vi "Init.vi"(8 "error in (no error)":errorcluster, 10 "Message":T1, 11 "Queue in":refnum<queue>) -> (0 "error out":errorcluster, 3 "Queue out":refnum<queue>)   [LabVIEW 2016]
uses:
  Controls/Message Structure.ctl
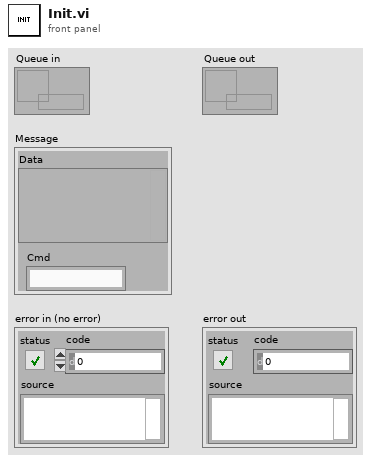
[diagram p1: front panel]
types:
  T1 = typedef "Message Structure.ctl" = cluster{"Data":variant, "Cmd":string}
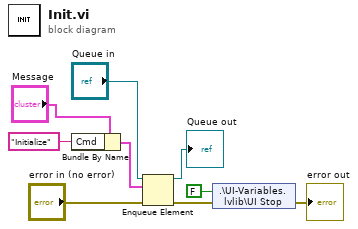
[diagram p0: block diagram]
diagram:
  n1 = Bundle By Name(cluster="Message", "Cmd"="Initialize") -> (w9:T1)
  n2 = Enqueue Element(queue="Queue in", element=w9, error in (no error)="error in (no error)") -> (queue out=→"Queue out":refnum<queue>, error out=w6:errorcluster)  [unwired: 1 in, 1 out]
  n3 = shared-variable ".\\UI-Variables.lvlib\\UI Stop"(FALSE ("UI Stop"), error in=w6) -> (error out=→"error out":errorcluster)
